vi "ArcadeDrive.vi"(10 "Turning":dbl, 11 "Power":dbl) -> (2 "Right_Motor":dbl, 3 "Left_Motor":dbl)   [LabVIEW 2018, in "ArgosLib.lvlib"]
uses:
  ArgosLib.lvlib
panel:
  # "ArcadeDrive"
  # "Makes Left and Right motor commands"
  # "Inputs"
  # "Outputs"
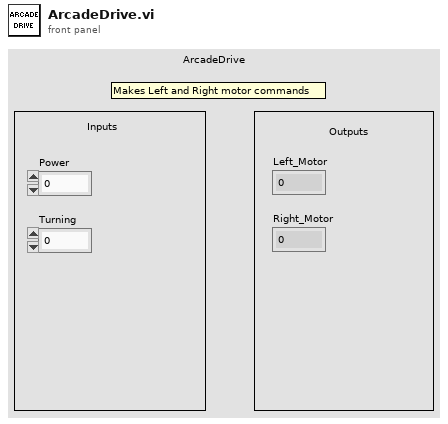
[diagram p1: front panel]
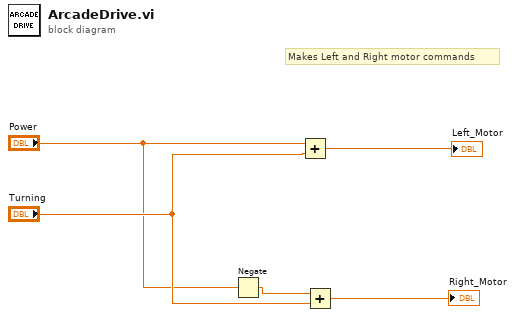
[diagram p0: block diagram]
diagram:
  # "Makes Left and Right motor commands"
  n1 = Negate(x="Power") -> (-x=w4:dbl)
  n2 = Add(x="Power", y="Turning") -> (x+y=→"Left_Motor":dbl)
  n3 = Add(x=w4, y="Turning") -> (x+y=→"Right_Motor":dbl)
